vi "Do.vi"(8 "error in (no error)":errorcluster, 10 "Actor in":refnum<class "Actor.lvclass">, 11 "Set Mode Msg":refnum<class "Set Mode Msg.lvclass">) -> (0 "error out":errorcluster, 2 "Actor out":refnum<class "Actor.lvclass">)   [LabVIEW 2016, in "CS++PPG.lvlib" / "Set Mode Msg.lvclass"]
doc: "This VI delivers the message to the actor by calling the appropriate method(s) on the actor."
uses:
  Set Mode Msg.lvclass
  <vilib>/ActorFramework/Actor/Actor.lvclass
  C:/User/Brand/LVP/CSPP-Dev/Packages/CSPP_Core/Actors/CS++PVMonitor Messages/CS++PVUpdate Msg/CS++PVUpdate Msg.lvclass
  CS++PPG/CS++PPG.lvclass
  C:/Program Files (x86)/National Instruments/LabVIEW 2016/vi.lib/ActorFramework/Actor/Actor.lvclass
  CSPP_Core/Actors/CS++PVMonitor Messages/CS++PVUpdate Msg/CS++PVUpdate Msg.lvclass/CS++PVUpdate Msg.ctl
  CSPP_Core/Classes/CS++ProcessVariables/ProcessVariable/PV.lvclass/PV.ctl
  Set Mode Msg.lvclass/Set Mode Msg.ctl
  CSPP_Core/Classes/CS++ProcessVariables/ProcessVariable/PV.lvclass
  CSPP_Core/Actors/CS++PVMonitor Messages/CS++PVUpdate Msg/CS++PVUpdate Msg.lvclass
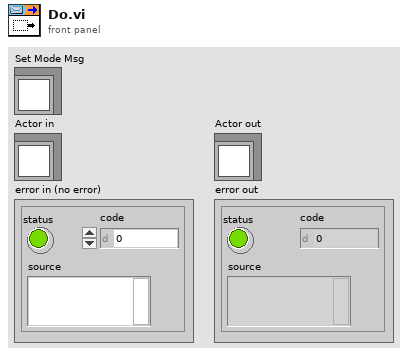
[diagram p1: front panel]
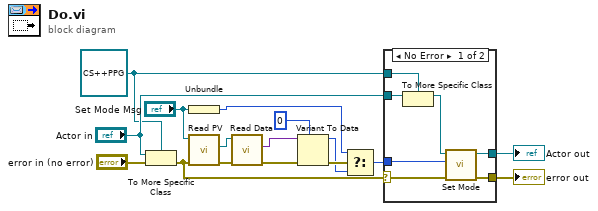
[diagram p0: block diagram]
diagram:
  w12 = refnum<class "CS++PPG.lvclass"> refnum ("Actor in")
  n1 = To More Specific Class(target class=w12, reference="Actor in", error in="error in (no error)") -> (error out=w3:errorcluster)  [unwired: 1 out]
  n2 = Unbundle ("Pre-Unbundler")("Set Mode Msg") -> (w1:u8)
  n3 = call "Read PV.vi"("error in (no error)"=w3, "CS++PVUpdate Msg in"="Set Mode Msg") -> ("error out"=w11:errorcluster, "PV"=w8:refnum<class "PV.lvclass">)  [unwired: 7 in, 1 out]
  n4 = call "Read Data.vi"("error in (no error)"=w11, "PV in"=w8) -> ("error out"=w6:errorcluster, "Data"=w7:variant)  [unwired: 7 in, 1 out]
  n5 = Variant To Data(error in=w6, type=u8 0 ("mode"), Variant=w7) -> (data=w5:u8, error out=w10:errorcluster)
  n6 = Select ("MainSelect")(t=w1, s=w10, f=w5) -> (s? t:f=w2:u8)
  n7 = case shown="No Error" w3 {
    selector: w3 -> [w21 w25]
    tunnel: [w23 w25] -> w15
    tunnel: [w22 w24] -> w14
    tunnel: "Actor in" -> [w20 w24]
    tunnel: w12 -> [w19 _]
    tunnel: w2 -> [w17 _]
    frame No Error {
      n8 = To More Specific Class(target class=w19, reference=w20) -> (specific class reference=w18:refnum<class "CS++PPG.lvclass">)  [unwired: 1 in, 1 out]
      n9 = call "Set Mode.vi"("error in (no error)"=w21, "mode"=w17, "CS++PPG in"=w18) -> ("error out"=w23:errorcluster, "CS++PPG out"=w22:refnum<class "CS++PPG.lvclass">)  [unwired: 7 in]
    }
    frame Error {
    }
  }
  "error out" <- w15
  "Actor out" <- w14
